vi "State_Machine.vi"(8 "error in (no error)":errorcluster caption="entrée d'erreur (pas d'erreur)", 11 "Get_Voltage en entrée":refnum<class "Nodon_Get_Product_ID.lvclass">) -> (0 "error out":errorcluster caption="sortie d'erreur", 2 "Json_String":string, 3 "Get_Voltage en sortie":refnum<class "Nodon_Get_Product_ID.lvclass">)   [LabVIEW 2020, in "Library Test.lvlib" / "Nodon_Get_Product_ID.lvclass"]
uses:
  Nodon_Get_Product_ID.lvclass
  C:/Users/ngarcin/OneDrive - Altyor/Standard TB/Class/Test/Nodon_Send_Command_UART/Nodon_Send_Command_UART.lvclass
  Nodon_Send_Command_UART.lvclass
  Nodon_Get_Product_ID.lvclass/Nodon_Get_Product_ID.ctl
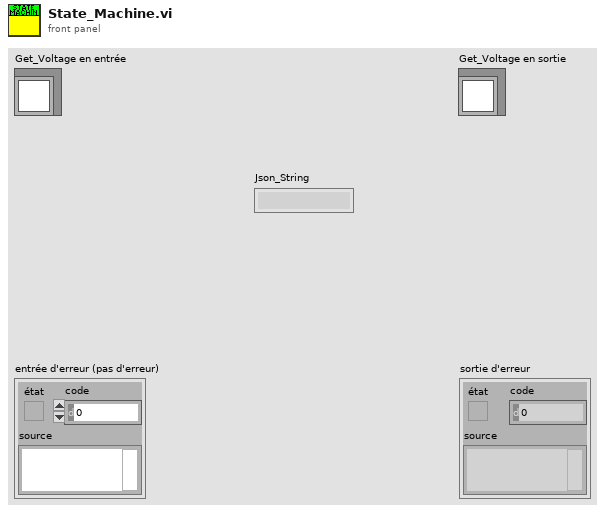
[diagram p1: front panel]
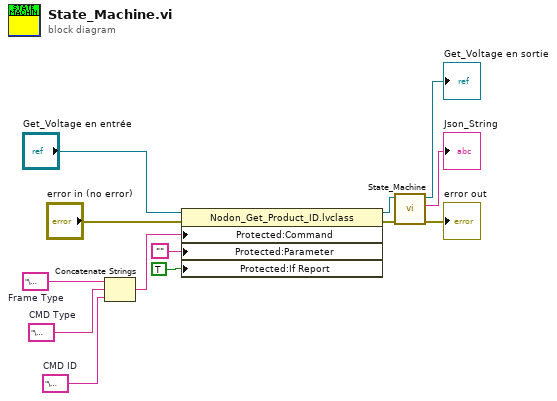
[diagram p0: block diagram]
diagram:
  w5 = "\u0000"  # Frame Type
  w4 = "\u0002"  # CMD ID
  w3 = "\u0002"  # CMD Type
  n1 = Concatenate Strings(w5, w3, w4) -> (w2:string)
  n2 = property class="Nodon_Get_Product_ID.lvclass"(reference="Get_Voltage en entrée", error in="error in (no error)", "Protected:Command"=w2, "Protected:Parameter"="", "Protected:If Report"=TRUE ("If Report")) -> (reference out=w8:refnum<class "Nodon_Get_Product_ID.lvclass">, error out=w6:errorcluster)
  n3 = call-parent "State_Machine.vi"("error in (no error)"=w6, "Send_Frame en entrée"=w8) -> ("error out"=→"error out":errorcluster, "Json_String"=→"Json_String":string, "Send_Frame en sortie"=→"Get_Voltage en sortie":refnum<class "Nodon_Get_Product_ID.lvclass">)  [unwired: 7 in]
